vi "Terminal_Global_ReferenceValue_Read.vi"   [LabVIEW 2014]
uses:
  Terminal-Global-ReferenceValues.vi
types:
  T1 = cluster{cluster{dbl, dbl}, cluster{dbl, dbl, dbl, dbl, dbl, dbl}, cluster{dbl, dbl}, cluster{dbl, dbl, dbl, dbl, dbl, dbl}}
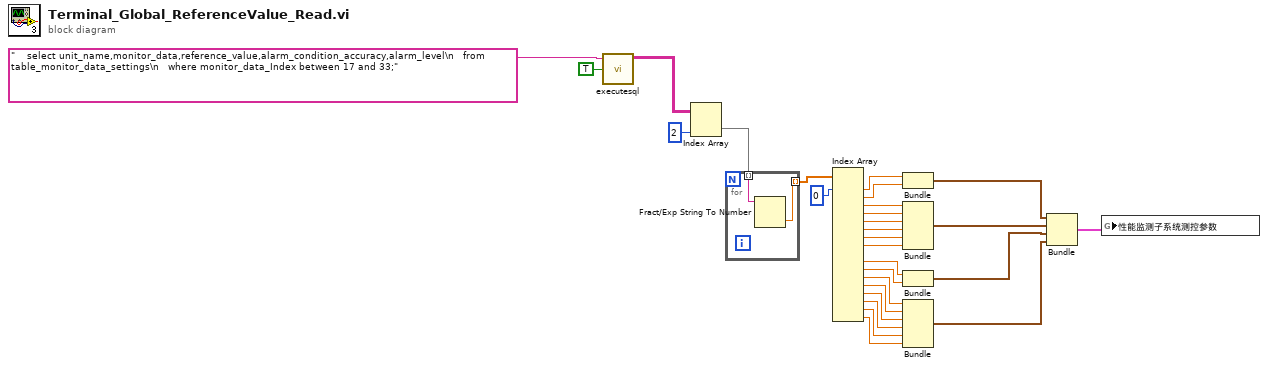
[diagram p0: block diagram]
diagram:
  n1 = call "executesql.vi"("Return Data (T)"=TRUE, "Command Text"="    select unit_name,monitor_data,reference_value,alarm_condition_accuracy,alarm_level\n   from table_monitor_data_settings\n   where monitor_data_Index between 17 and 33;") -> ("Data"=w26:string[][])  [unwired: 5 in, 1 out]
  n2 = Index Array(array=w26, index (col)=2 ("禁用的索引 (列)")) -> (element=w21:string[])  [unwired: 1 in]
  n3 = for {
    tunnel: w21 -> [w30] mode=indexing
    tunnel: [w29] -> w20 mode=indexing
    n4 = Fract/Exp String To Number(string=w30) -> (number=w29:dbl)  [unwired: 3 in, 1 out]
  }
  n5 = Index Array(array=w20, index #1=0 ("索引")) -> (element #1=w23:dbl, element #2=w22:dbl, element #3=w19:dbl, element #4=w18:dbl, element #5=w17:dbl, element #6=w16:dbl, element #7=w15:dbl, element #8=w14:dbl, element #10=w13:dbl, element #11=w12:dbl, element #12=w11:dbl, element #13=w10:dbl, element #14=w9:dbl, element #15=w8:dbl, element #16=w7:dbl, element #17=w6:dbl)  [unwired: 16 in, 1 out]
  n6 = Bundle(w23, w22) -> (w5:cluster{dbl, dbl})  [unwired: 1 in]
  n7 = Bundle(w19, w18, w17, w16, w15, w14) -> (w4:cluster{dbl, dbl, dbl, dbl, dbl, dbl})  [unwired: 1 in]
  n8 = Bundle(w13, w12) -> (w3:cluster{dbl, dbl})  [unwired: 1 in]
  n9 = Bundle(w11, w10, w9, w8, w7, w6) -> (w2:cluster{dbl, dbl, dbl, dbl, dbl, dbl})  [unwired: 1 in]
  n10 = Bundle(w5, w4, w3, w2) -> (w1:T1)  [unwired: 1 in]
  n11 = global write "Terminal-Global-ReferenceValues.vi" "性能监测子系统测控参数"(w1) -> ()
